vi "Save LFO Report.vi"(4 "Raw Data Path":path, 6 "Bridgewire 2 No-Fire":refnum<vi>, 7 "Bridgewire 1 No-Fire":refnum<vi>, 8 "error in (no error)":errorcluster, 9 "Results Table":string[][](array[string]), 10 "Serial Number":string="LFO Electrical Test Results", 11 "Part Number":string="LFO Electrical Test Results") -> (0 "error out":errorcluster)   [LabVIEW 2018]
uses:
  <vilib>/Utility/NIReport.llb/NI_report.lvclass
  <vilib>/Utility/NIReport.llb/Report Type.ctl
  <vilib>/addons/_office/_exclsub.llb/font.ctl
  <vilib>/Utility/NIReport.llb/HTML Report Image Alignment.ctl
  <vilib>/addons/_office/word.llb/Word Easy Table (str).vi
  <vilib>/addons/_office/NI_ReportGenerationToolkit.lvlib
  <vilib>/Utility/NIReport.llb/NI_ReportGenerationCore.lvlib
  <vilib>/Utility/NIReport.llb/Word/NI_Word.lvclass
panel:
  out "appended path":path
  out "report out":refnum<class "NI_report.lvclass">
  in  "row headers":string[](array[string])=["Min", "Max", "Measured"]
  in  "Column Headers":string[](array[string])=["BW1\nResistance\n(Ohms)", "BW2\nResistance\n(Ohms)", "BW1\nNo-Fire", "BW2\nNo-Fire", "BW1\nDielectric Strength\n(uA)", "BW2\nDielectric Strength\n(uA)", "BW1\nInsulation Resistance\n(Megaohms)", "BW2\nInsulation Resistance\n(Megaohms)"]
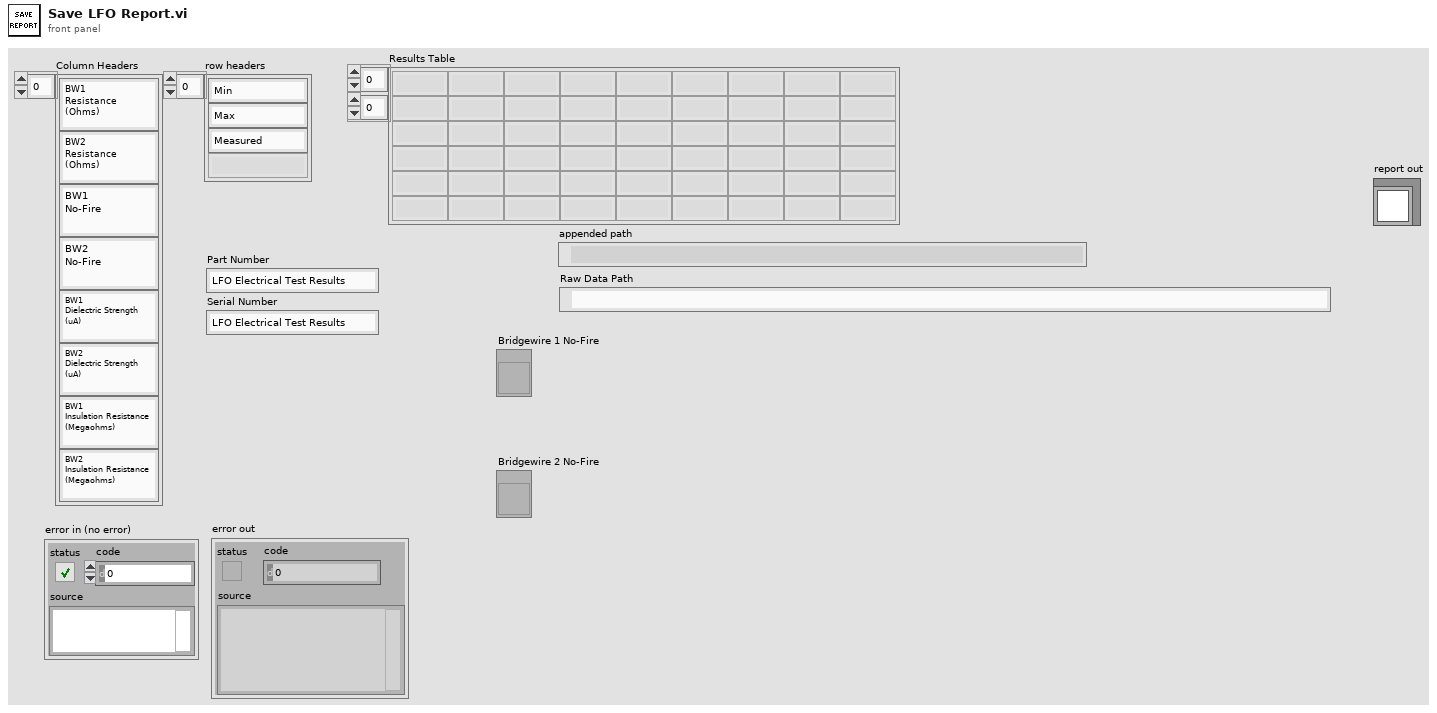
[diagram p1: front panel]
types:
  T1 = typedef "NI_ReportGenerationCore.lvlib/HTML Report Image Alignment.ctl" = enum16{"(default)", "LEFT", "RIGHT", "TOP", "TEXTTOP", "MIDDLE", "ABSMIDDLE", "BASELINE", "BOTTOM", "ABSBOTTOM"}
  T2 = typedef "NI_ReportGenerationToolkit.lvlib/font.ctl" = cluster{"font name":string, "font size":dbl, "bold":u16, "italic":u16, "underline":u16, "strike through":u16, "font color":u32}
  T3 = typedef "NI_ReportGenerationCore.lvlib/Report Type.ctl" = enum16{"HTML", "Word", "Excel"}
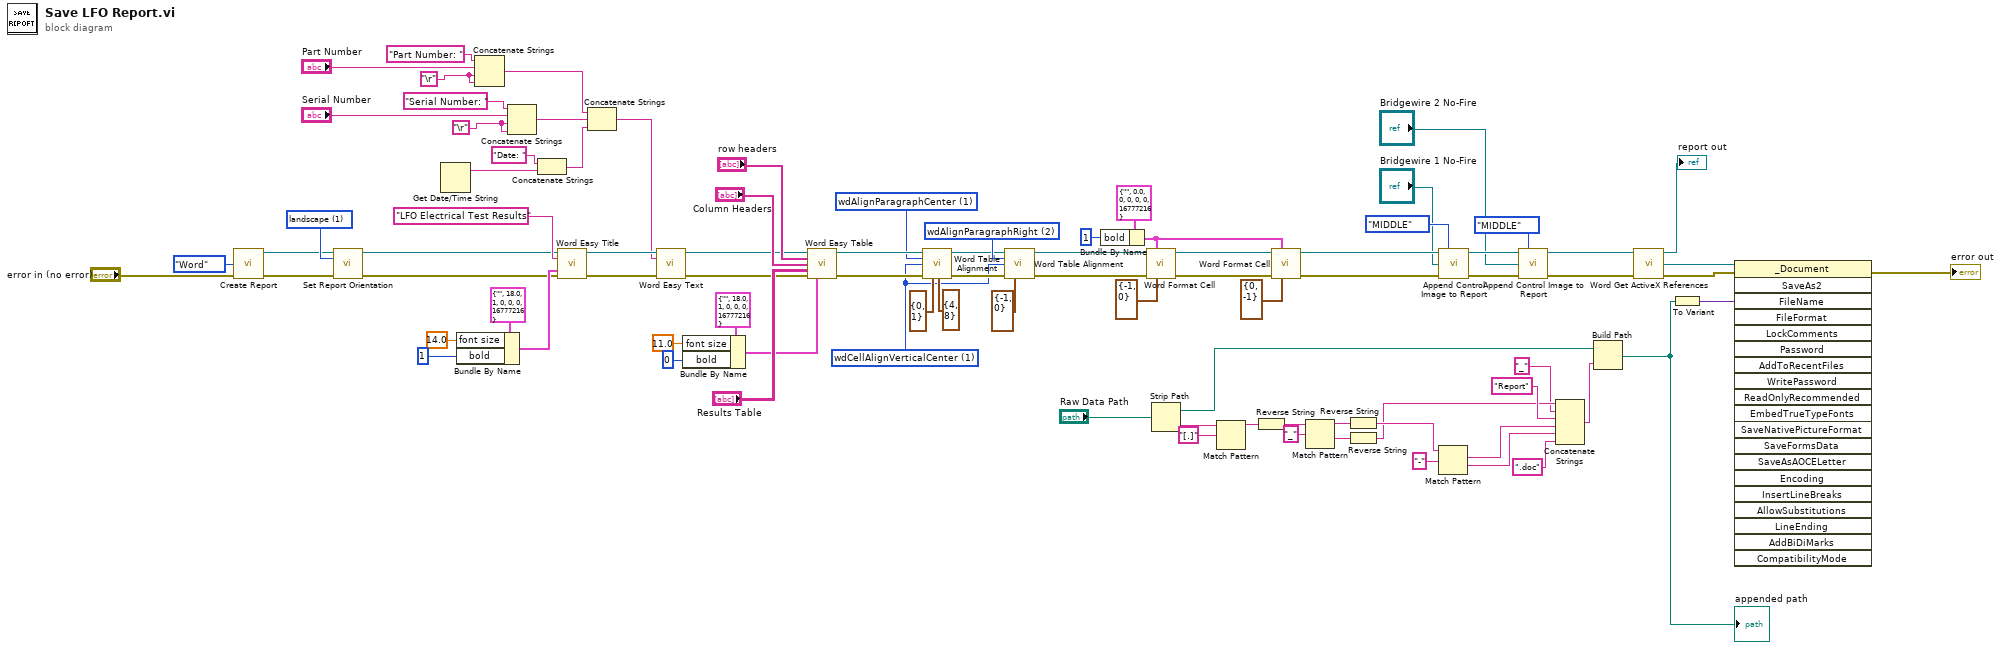
[diagram p0: block diagram]
diagram:
  w49 = 2 items=["wdAlignParagraphLeft"=0, "wdAlignParagraphCenter"=1, "wdAlignParagraphRight"=2, "wdAlignParagraphJustify"=3, "wdAlignParagraphDistribute"=4, "wdAlignParagraphJustifyMed"=5, "wdAlignParagraphJustifyHi"=7, "wdAlignParagraphJustifyLow"=8] ("horizontal alignment (left)")
  w37 = 1 items=["wdCellAlignVerticalTop"=0, "wdCellAlignVerticalCenter"=1, "wdCellAlignVerticalBottom"=3] ("vertical alignment (top)")
  w54 = 1 items=["wdAlignParagraphLeft"=0, "wdAlignParagraphCenter"=1, "wdAlignParagraphRight"=2, "wdAlignParagraphJustify"=3, "wdAlignParagraphDistribute"=4, "wdAlignParagraphJustifyMed"=5, "wdAlignParagraphJustifyHi"=7, "wdAlignParagraphJustifyLow"=8] ("horizontal alignment (left)")
  w56 = 1 items=["portrait", "landscape"] ("orientation (portrait)")
  w72 = "\r"
  w73 = "\r"
  n1 = call <vilib>:"Create Report.vi"("report type"=Report_Type."Word", "error in (no error)"="error in (no error)") -> ("report out"=w28:refnum<class "NI_report.lvclass">, "error out"=w58:errorcluster)  [unwired: 12 in]
  n2 = call-dynamic "Set Report Orientation.vi"("report in"=w28, "orientation (portrait)"=w56, "error in (no error)"=w58) -> ("report out"=w59:refnum<class "NI_report.lvclass">, "error out"=w57:errorcluster)  [unwired: 11 in]
  n3 = Get Date/Time String() -> (date string=w68:string)  [unwired: 3 in, 1 out]
  n4 = Bundle By Name(cluster=T2 {"font name"="", "font size"=18.0, "bold"=1, "italic"=0, "underline"=0, "strike through"=0, "font color"=16777216} ("font"), "font size"=14.0, "bold"=u16 1) -> (w83:T2)
  n5 = Concatenate Strings("Part Number: " ("title"), "Part Number", w73, w73) -> (w67:string)
  n6 = Concatenate Strings("Serial Number: " ("title"), "Serial Number", w72, w72) -> (w66:string)
  n7 = Concatenate Strings("Date: " ("title"), w68) -> (w65:string)
  n8 = call <vilib>:"Word Easy Title.vi"("report in"=w59, "title"="LFO Electrical Test Results", "font"=w83, "error in (no error)"=w57) -> ("report out"=w78:refnum<class "NI_report.lvclass">, "error out"=w79:errorcluster)  [unwired: 9 in, 1 out]
  n9 = Concatenate Strings(w67, w66, w65) -> (w64:string)
  n10 = call <vilib>:"Word Easy Text.vi"("report in"=w78, "text"=w64, "error in (no error)"=w79) -> ("report out"=w77:refnum<class "NI_report.lvclass">, "error out"=w76:errorcluster)  [unwired: 10 in, 1 out]
  n11 = Bundle By Name(cluster=T2 {"font name"="", "font size"=18.0, "bold"=1, "italic"=0, "underline"=0, "strike through"=0, "font color"=16777216} ("font"), "font size"=11.0, "bold"=u16 0) -> (w61:T2)
  n12 = call-poly <vilib>:"Word Easy Table.vi"("report in"=w77, "row headers"="row headers", "column headers"="Column Headers", "data"="Results Table", "error in (no error)"=w76, "font"=w61) -> ("report out"=w55:refnum<class "NI_report.lvclass">, "error out"=w53:errorcluster)  [unwired: 7 in, 1 out]
  n13 = call <vilib>:"Word Table Alignment.vi"("report in"=w55, "horizontal alignment (left)"=w54, "vertical alignment (top)"=w37, "error in (no error)"=w53, "start (-1, -1)"=cluster{"start row":i32, "start column":i32} {"start row"=0, "start column"=1}, "end (-1, -1)"=cluster{"end row":i32, "end column":i32} {"end row"=4, "end column"=8}) -> ("report out"=w48:refnum<class "NI_report.lvclass">, "error out"=w47:errorcluster)  [unwired: 8 in]
  n14 = call <vilib>:"Word Table Alignment.vi"("report in"=w48, "horizontal alignment (left)"=w49, "vertical alignment (top)"=w37, "error in (no error)"=w47, "start (-1, -1)"=cluster{"start row":i32, "start column":i32} {"start row"=-1, "start column"=0}) -> ("report out"=w46:refnum<class "NI_report.lvclass">, "error out"=w45:errorcluster)  [unwired: 9 in]
  n15 = Bundle By Name(cluster=T2 {"font name"="", "font size"=0.0, "bold"=0, "italic"=0, "underline"=0, "strike through"=0, "font color"=16777216} ("font"), "bold"=u16 1) -> (w38:T2)
  n16 = call <vilib>:"Word Format Cell.vi"("report in"=w46, "font"=w38, "error in (no error)"=w45, "start (-1, -1)"=cluster{"start row":i32, "start column":i32} {"start row"=-1, "start column"=0}) -> ("report out"=w40:refnum<class "NI_report.lvclass">, "error out"=w39:errorcluster)  [unwired: 10 in]
  n17 = Strip Path(path="Raw Data Path") -> (stripped path=w24:path, name=w21:string)
  n18 = Match Pattern(string=w21, regular expression="[.]") -> (before substring=w15:string)  [unwired: 1 in, 3 out]
  n19 = Reverse String(1:w15) -> (0:w14:string)
  n20 = call <vilib>:"Word Format Cell.vi"("report in"=w40, "font"=w38, "error in (no error)"=w39, "start (-1, -1)"=cluster{"start row":i32, "start column":i32} {"start row"=0, "start column"=-1}) -> ("report out"=w36:refnum<class "NI_report.lvclass">, "error out"=w35:errorcluster)  [unwired: 10 in]
  n21 = Match Pattern(string=w14, regular expression="_") -> (before substring=w13:string, after substring=w12:string)  [unwired: 1 in, 2 out]
  n22 = Reverse String(1:w13) -> (0:w11:string)
  n23 = Reverse String(1:w12) -> (0:w10:string)
  n24 = Match Pattern(string=w11, regular expression="-") -> (match substring=w17:string, after substring=w18:string)  [unwired: 1 in, 2 out]
  n25 = call-dynamic "Append Control Image to Report.vi"("report in"=w36, "alignment (default)"=HTML_Report_Image_Alignment."MIDDLE", "ctrl reference"="Bridgewire 1 No-Fire", "error in (no error)"=w35) -> ("report out"=w4:refnum<class "NI_report.lvclass">, "error out"=w3:errorcluster)  [unwired: 8 in, 2 out]
  n26 = call-dynamic "Append Control Image to Report.vi"("report in"=w4, "alignment (default)"=HTML_Report_Image_Alignment."MIDDLE", "ctrl reference"="Bridgewire 2 No-Fire", "error in (no error)"=w3) -> ("report out"=w32:refnum<class "NI_report.lvclass">, "error out"=w31:errorcluster)  [unwired: 8 in, 2 out]
  n27 = Concatenate Strings(w10, "_" ("string"), "Report" ("string"), w17, w18, ".doc" ("string")) -> (w22:string)
  n28 = Build Path(base path=w24, name or relative path=w22) -> (appended path=w8:path)
  "appended path" <- w8
  n29 = call <vilib>:"Word Get ActiveX References.vi"("report in"=w32, "error in (no error)"=w31) -> ("report out"=→"report out":refnum<class "NI_report.lvclass">, "Word._Document"=w29:refnum<k7>, "error out"=w30:errorcluster)  [unwired: 7 in, 4 out]
  n30 = To Variant(anything=w8) -> (Variant=w27:variant)
  n31 = invoke class="_Document" method="SaveAs2"(reference=w29, error in=w30, "FileName"=w27) -> (error out=→"error out":errorcluster)  [unwired: 17 in, 19 out]
